vi "AE - Bluetooth Battery.vi"(8 "error in (no error)":errorcluster, 11 "Wiimote":u8) -> (0 "error out":errorcluster, 2 "Battery Raw":u8, 3 "Battery Level":dbl)   [LabVIEW 2011]
uses:
  AE Cores/AE - Bluetooth Enum.ctl
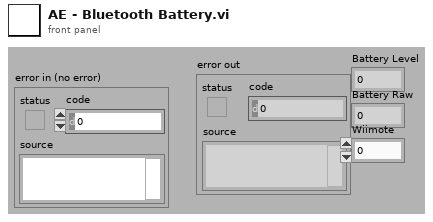
[diagram p1: front panel]
types:
  T1 = typedef "AE - Bluetooth Enum.ctl" = enum16{"Initialise", "Pair All Wiimotes", "Connect All Wiimotes", "Set Rumble", "Set LED", "Get Button + Acc Data", "Get IR Data", "Get Battery", "Get Wiimote Reference", "Reorder Wiimotes", "devReport"}
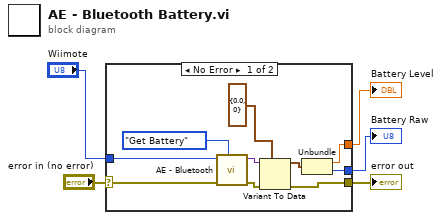
[diagram p0: block diagram]
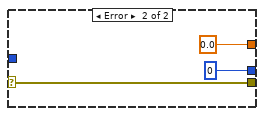
[diagram p2: hidden frame]
diagram:
  n1 = case shown="No Error" "error in (no error)" {
    selector: "error in (no error)" -> [w14 w18]
    tunnel: [w9 w18] -> w4
    tunnel: [w8 0.0] -> w3
    tunnel: [w7 u8 0] -> w2
    tunnel: "Wiimote" -> [w6 _]
    frame No Error {
      n2 = call "AE - Bluetooth.vi"("Enum"=AE_-_Bluetooth_Enum."Get Battery", "error in (no error)"=w14, "Variant In"=w6) -> ("error out"=w10:errorcluster, "Variant Out"=w13:variant)  [unwired: 6 in, 1 out]
      n3 = Variant To Data(error in=w10, type=cluster{dbl, u8} {0.0, 0}, Variant=w13) -> (data=w11:cluster{dbl, u8}, error out=w9:errorcluster)
      n4 = Unbundle(w11) -> (w8:dbl, w7:u8)
    }
    frame Error {
    }
  }
  "error out" <- w4
  "Battery Level" <- w3
  "Battery Raw" <- w2
